vi "Examen 1.vi"() -> ()   [LabVIEW 2020]
uses:
  <vilib>/numeric/Random Number (Range) U64.vi
  <vilib>/numeric/sub_Random U32.vi
panel:
  out "Waveform Chart":dbl[][](graph)
  in  "Detener":bool
  out "Sobre el límite máximo":i32
  out "Histeresis":bool
  out "Dentro del rango":bool
  out "Valor Actual":u64
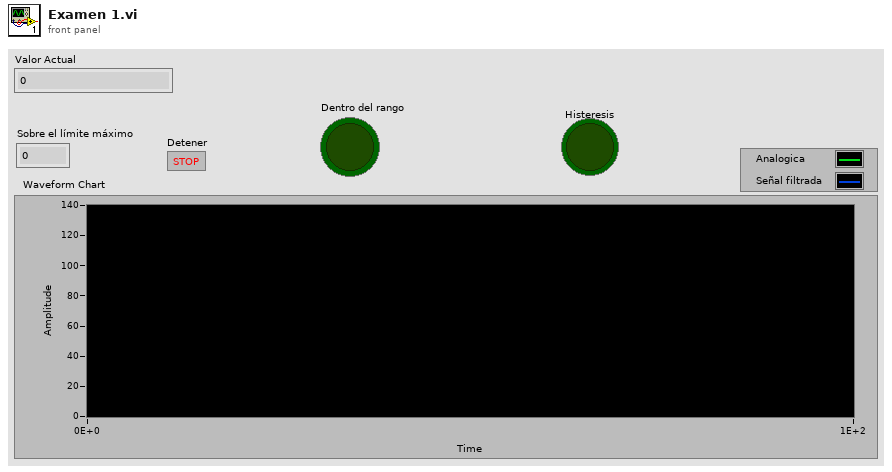
[diagram p1: front panel]
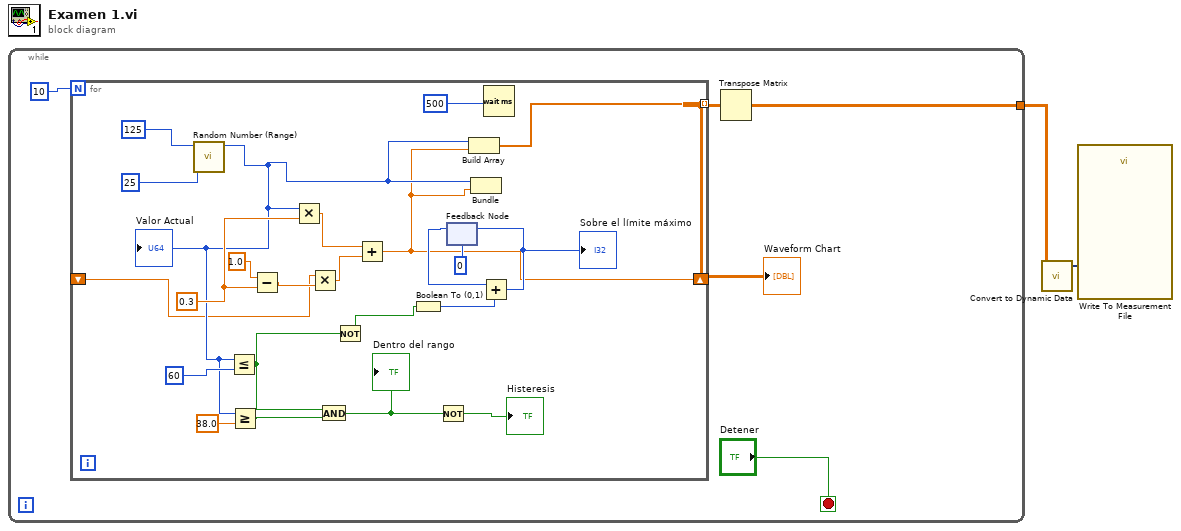
[diagram p0: block diagram]
diagram:
  n1 = while {
    tunnel: [w3] -> w2
    stop <- "Detener" stop-if-true
    n2 = for {
      N: 10 -> [_]
      tunnel: [w7] -> w4 mode=indexing
      shift-right: [w8] -> _
      shift-left: _ -> [w9]
      w27 = 0.3 ("y")
      n3 = call-poly <vilib>:"Random Number (Range).vi"("lower bound (0)"=u64 25, "upper bound (100)"=u64 125) -> ("number"=w10:u64)  [unwired: 9 in]
      "Valor Actual" <- w10
      n4 = Less Or Equal?(x=w10, y=u64 60) -> (x <= y?=w19:bool)
      n5 = Greater Or Equal?(x=w10, y=38.0) -> (x >= y?=w20:bool)
      n6 = Subtract(x=1.0, y=w27) -> (x-y=w25:dbl)
      n7 = Multiply(x=w10, y=w27) -> (x*y=w24:dbl)
      n8 = Multiply(x=w9, y=w25) -> (x*y=w23:dbl)
      n9 = And(x=w19, y=w20) -> (x .and. y?=w18:bool)
      "Dentro del rango" <- w18
      n10 = Not(x=w19) -> (.not. x?=w16:bool)
      n11 = Add(x=w24, y=w23) -> (x+y=w8:dbl)
      n12 = Boolean To (0,1)(Boolean=w16) -> (0, 1=w15:i16)
      n13 = Not(x=w18) -> (.not. x?=→"Histeresis":bool)
      n14 = feedback #1(0) -> (w12:i32)
      n15 = Build Array(w10, w8) -> (w7:dbl[])
      n16 = Bundle("number"=w10, w8) -> ()  [unwired: 1 in, 1 out]
      n17 = Add(x=w12, y=w15) -> (x+y=w13:i32)
      "Sobre el límite máximo" <- w13
      n18 = feedback-in #1(w13) -> ()
      n19 = Wait (ms)(milliseconds to wait=u32 500) -> ()  [unwired: 1 out]
    }
    "Waveform Chart" <- w4
    n20 = Transpose Matrix(1:w4) -> (0:w3:dbl[][])
  }
  n21 = call "Convert to Dynamic Data"("2D Array"=w2) -> ("Dynamic Data Type"=w1:dynamicdata)  [unwired: 3 in]
  n22 = call "Write To Measurement File"("Signals"=w1) -> ()  [unwired: 16 in, 3 out]
